vi "Create Cal Sweep File.vi"(0 "Sweep Name":string, 5 "Grid":T1, 11 "error in (no error)":errorcluster) -> (4 "Sweep File Path":path, 15 "error out":errorcluster)   [LabVIEW 2023, in "RFFixtureCharact.RFPM.lvlib" / "Vector 18GHz Path.lvclass"]
uses:
  Vector 18GHz Path.lvclass
  Path Groups/Vector Path Group/Type Definitions/Sweep.ctl
  C:/rfcal/AuxTools/STSRFFixtureCharactUtility/Source/Code Modules/Dependencies/NationalInstruments.RFCalibration.SweepSettingsUtility.dll
  Dependencies/NationalInstruments.RFCalibration.SweepSettingsUtility.dll
  Instruments/Cal Standard/Cal Standard Base/Cal Standard Base.lvclass
  Vector 18GHz Path.lvclass/Vector 18GHz Path.ctl
  Instruments/Cal Standard/Cal Standard Factory/Cal Standard Factory.lvclass
  Public/RFFixtureCharact.Public.lvlib
  Path Groups/Vector Path Group/Vector 18GHz Path Group.lvclass
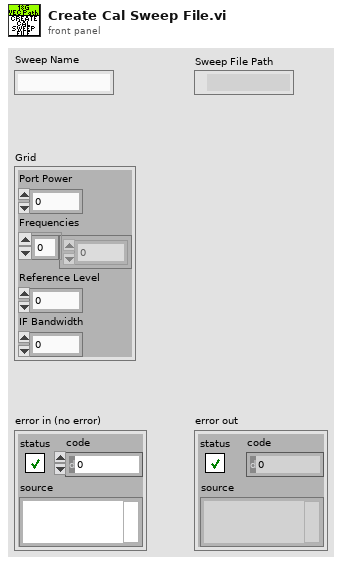
[diagram p1: front panel]
types:
  T1 = typedef "RFFixtureCharact.RFPM.lvlib/Vector 18GHz Path Group.lvclass/Sweep.ctl" = cluster{"Port Power":dbl, "Frequencies":dbl[], "Reference Level":dbl, "IF Bandwidth":dbl}
  T2 = enum16{"open", "replace", "create", "open or create", "replace or create", "replace or create with confirmation"}
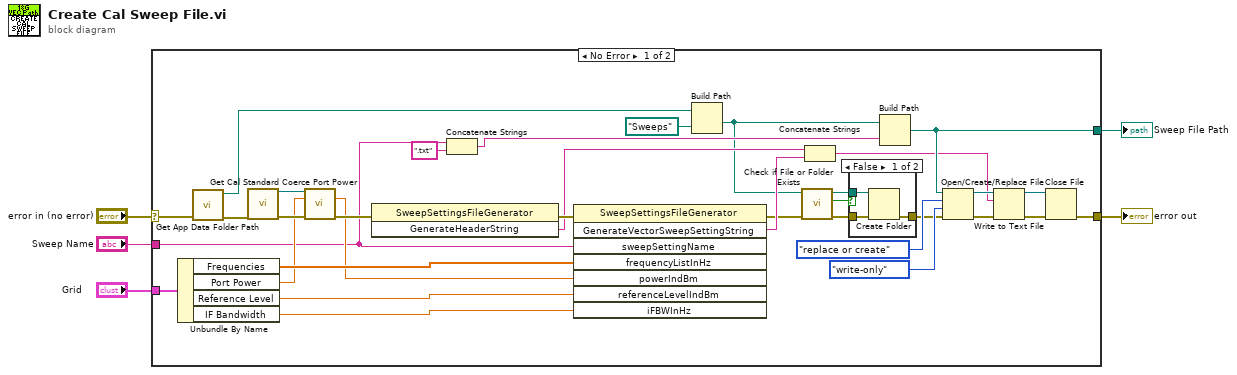
[diagram p0: block diagram]
diagram:
  n1 = case shown="No Error" "error in (no error)" {
    selector: "error in (no error)" -> [w12 w44]
    tunnel: [w27 w44] -> w4
    tunnel: "Grid" -> [w38 _]
    tunnel: [w32 _] -> w3
    tunnel: "Sweep Name" -> [w6 _]
    frame No Error {
      n2 = Unbundle By Name(w38) -> ("Frequencies"=w37:dbl[], "Port Power"=w14:dbl, "Reference Level"=w36:dbl, "IF Bandwidth"=w7:dbl)
      n3 = call "Get App Data Folder Path.vi"("error in (no error)"=w12) -> ("error out"=w11:errorcluster, "Temp Folder Path"=w10:path)  [unwired: 9 in]
      n4 = call "Get Cal Standard.vi"("error in (no error)"=w11) -> ("Cal Standard Base out"=w15:refnum<class "Cal Standard Base.lvclass">, "error out"=w17:errorcluster)  [unwired: 12 in, 1 out]
      n5 = call-dynamic "Coerce Port Power.vi"("Cal Standard Base in"=w15, "Port Power"=w14, "error in (no error)"=w17) -> ("Coerced Port Power"=w13:dbl, "error out"=w16:errorcluster)  [unwired: 10 in, 1 out]
      n6 = invoke class="SweepSettingsFileGenerator" method="GenerateHeaderString"(error in=w16) -> (error out=w39:errorcluster, "GenerateHeaderString"=w35:string)  [unwired: 2 in, 1 out]
      n7 = Concatenate Strings(w6, ".txt" ("string")) -> (w18:string)
      n8 = invoke class="SweepSettingsFileGenerator" method="GenerateVectorSweepSettingString"(error in=w39, "sweepSettingName"=w6, "frequencyListInHz"=w37, "powerIndBm"=w13, "referenceLevelIndBm"=w36, "iFBWInHz"=w7) -> (error out=w24:errorcluster, "GenerateVectorSweepSettingString"=w34:string)  [unwired: 2 in, 6 out]
      n9 = Build Path(base path=w10, name or relative path=path "Sweeps" ("base path")) -> (appended path=w8:path)
      n10 = call <vilib>:"Check if File or Folder Exists.vi"("error in (no error)"=w24, "path"=w8) -> ("error out"=w23:errorcluster, "file or folder exists?"=w22:bool, "dup path"=w21:path)  [unwired: 7 in]
      n11 = Concatenate Strings(w35, w34) -> (w29:string)
      n12 = case shown="False" w22 {
        tunnel: w23 -> [w42 w43]
        tunnel: w21 -> [w41 _]
        tunnel: [w40 w43] -> w20
        frame False {
          n13 = Create Folder(path (use dialog)=w41, error in=w42) -> (error out=w40:errorcluster)  [unwired: 1 in, 2 out]
        }
        frame True {
        }
      }
      n14 = Build Path(base path=w8, name or relative path=w18) -> (appended path=w32:path)
      n15 = Open/Create/Replace File(file path (use dialog)=w32, error in=w20, operation (0:open)=T2."replace or create", access (0:read/write)=enum16{"read/write", "read-only", "write-only"}."write-only") -> (refnum out=w30:refnum<file>, error out=w33:errorcluster)  [unwired: 2 in, 1 out]
      n16 = Write to Text File(file (use dialog)=w30, text=w29, error in=w33) -> (refnum out=w26:refnum<file>, error out=w28:errorcluster)  [unwired: 1 in, 1 out]
      n17 = Close File(refnum=w26, error in=w28) -> (error out=w27:errorcluster)  [unwired: 1 out]
    }
    frame Error {
    }
  }
  "error out" <- w4
  "Sweep File Path" <- w3
